vi "Store CVT Session.vi"(7 "Action":enum16{"Read", "Write"}(ring), 11 "CVT Session In":T1) -> (3 "CVT Session Out":refnum<data-value>)   [LabVIEW 2016, in "Controller.lvlib" / "gController.lvclass"]
uses:
  gController.lvclass
  <vilib>/MSR Consulting, LLC/General Reuse/Session APIs/_Session Fwk/Typedefs/Session Handle.ctl
  <vilib>/MSR Consulting, LLC/General Reuse/Session APIs/_Session Fwk/Session - Root.lvclass
  <vilib>/MSR Consulting, LLC/General Reuse/Session APIs/CVT/CVT.lvclass
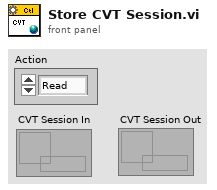
[diagram p1: front panel]
types:
  T1 = typedef "Session - Root.lvclass/Session Handle.ctl" = refnum<data-value>
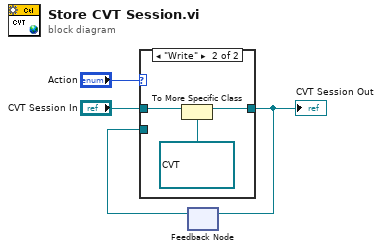
[diagram p0: block diagram]
diagram:
  n1 = feedback #1() -> (w1:refnum<data-value>)  [unwired: 1 in]
  n2 = case shown="\"Write\"" "Action" {
    tunnel: "CVT Session In" -> [_ w8]
    tunnel: [w5 w6] -> w2
    tunnel: w1 -> [w5 _]
    frame "Read", Default {
    }
    frame "Write" {
      n3 = To More Specific Class(target class=refnum<data-value> refnum, reference=w8) -> (specific class reference=w6:refnum<data-value>)  [unwired: 1 in, 1 out]
    }
  }
  "CVT Session Out" <- w2
  n4 = feedback-in #1(w2) -> ()
